vi "SeqMgr.Parse Set Function.vi"() -> ()   [LabVIEW 2024, in "EQMF.lvlib" / "SeqMgr.lvlib"]
uses:
  SeqMgr.lvlib
panel:
  out "error":errorcluster
  out "Step":string[](array[string])
  in  "Text":string
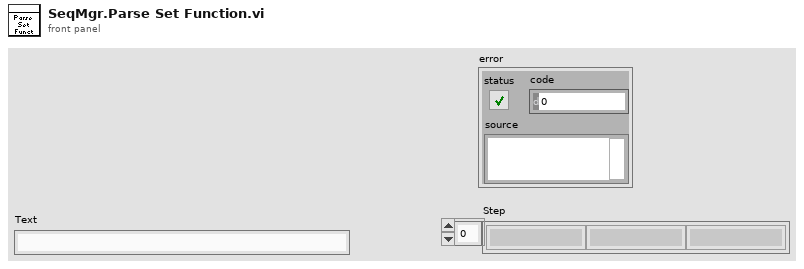
[diagram p1: front panel]
types:
  T1 = cluster{"Funct":string, "Params":string[], "Text":string}
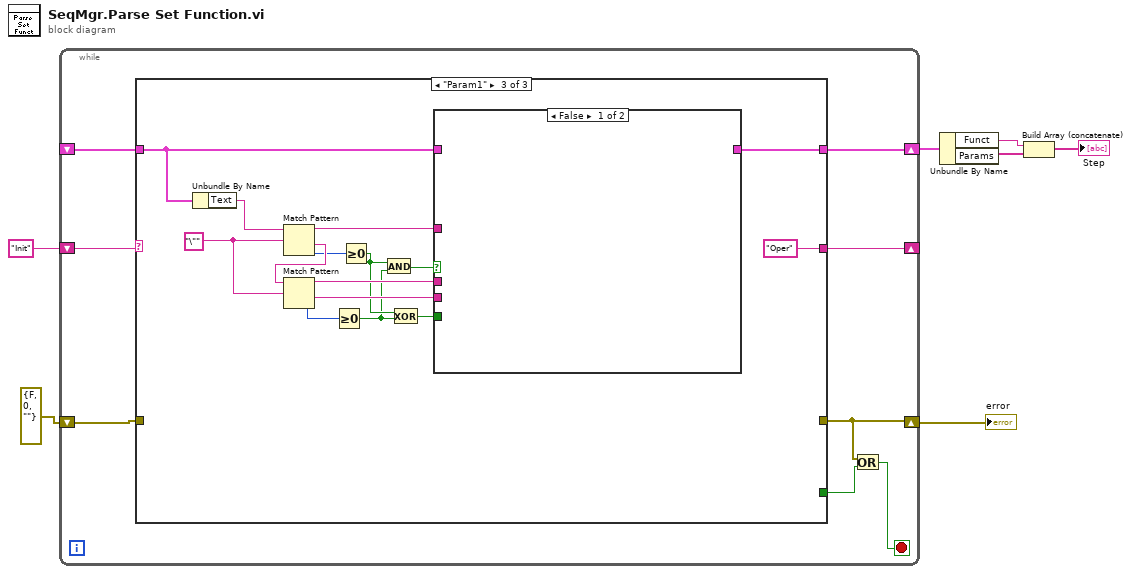
[diagram p0: block diagram]
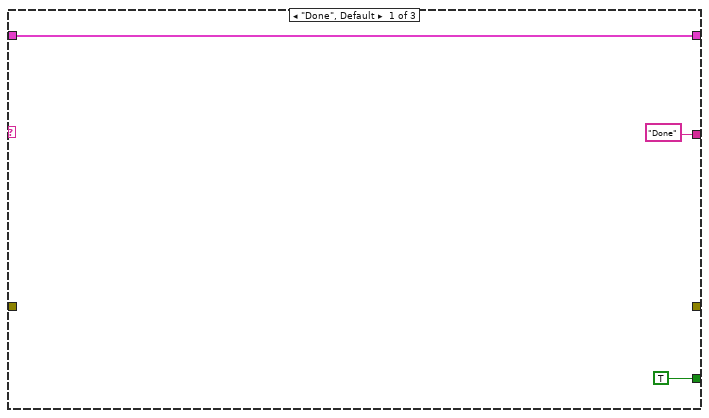
[diagram p2: hidden frame]
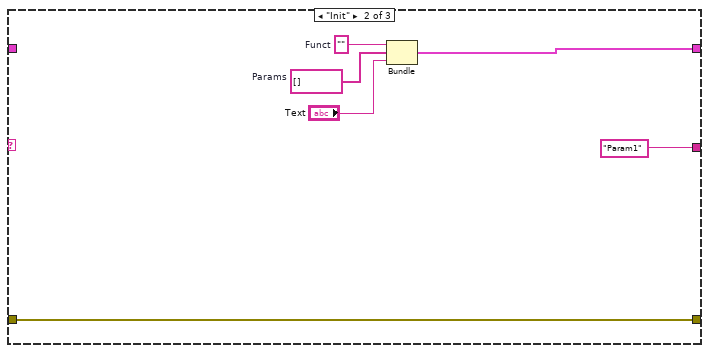
[diagram p3: hidden frame]
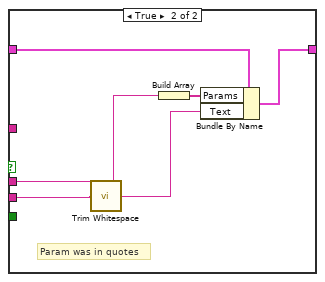
[diagram p4: hidden frame]
diagram:
  n1 = while {
    shift-right: [w14] -> w5
    shift-left: _ -> [w12]
    shift-right: [w13] -> _
    shift-left: "Init" -> [w15]
    shift-right: [w8] -> w1
    shift-left: errorcluster {"status"=FALSE, "code"=0, "source"=""} ("error constant") -> [w11]
    stop <- w9 stop-if-true
    n2 = case shown="\"Param1\"" w15 {
      tunnel: [w16 w23 w30] -> w14
      tunnel: ["Done" "Param1" "Oper"] -> w13
      tunnel: [TRUE _ _] -> w10
      tunnel: w12 -> [w16 _ w31]
      tunnel: w11 -> [_ w20 _]
      tunnel: [_ w20 _] -> w8
      frame "Done", Default {
      }
      frame "Init" {
        w22 = ""  # Funct
        w21 = string[] []  # Params
        n3 = Bundle("Funct"=w22, "Params"=w21, "Text"="Text") -> (w23:T1)  [unwired: 1 in]
      }
      frame "Param1" {
        w38 = "\""
        n4 = Unbundle By Name(w31) -> ("Text"=w37:string)
        n5 = Match Pattern(string=w37, regular expression=w38) -> (before substring=w36:string, after substring=w39:string, offset past match=w34:i32)  [unwired: 1 in, 1 out]
        n6 = Match Pattern(string=w39, regular expression=w38) -> (before substring=w35:string, after substring=w28:string, offset past match=w33:i32)  [unwired: 1 in, 1 out]
        n7 = Greater Or Equal To 0?(x=w33) -> (x >= 0?=w26:bool)
        n8 = Greater Or Equal To 0?(x=w34) -> (x >= 0?=w27:bool)
        n9 = And(x=w27, y=w26) -> (x .and. y?=w32:bool)
        n10 = Exclusive Or(1:w26, 2:w27) -> (0:w25:bool)
        n11 = case shown="False" w32 {
          tunnel: w36 -> [_ _]
          tunnel: w35 -> [_ w43]
          tunnel: w31 -> [_ w45]
          tunnel: [_ w42] -> w30
          tunnel: w28 -> [_ w41]
          tunnel: w25 -> [_ _]
          frame False {
          }
          frame True {
            # "Param was in quotes"
            n12 = call <vilib>:"Trim Whitespace.vi"("string"=w41) -> ("trimmed string"=w40:string)  [unwired: 1 in]
            n13 = Build Array(w43) -> (w44:string[])
            n14 = Bundle By Name(cluster=w45, "Params"=w44, "Text"=w40) -> (w42:T1)
          }
        }
      }
    }
    n15 = Or(x=w8, y=w10) -> (x .or. y?=w9:bool)
  }
  "error" <- w1
  n16 = Unbundle By Name(w5) -> ("Funct"=w4:string, "Params"=w3:string[])
  n17 = Build Array (concatenate)(w4, w3) -> (→"Step":string[])
